vi "Button To Toggle Vr4.vi"(1 "InValue":bool, 2 "Action":enum16{"onPress", "onRelease", "Both"}(ring)) -> (0 "Result":bool)   [LabVIEW 2012]
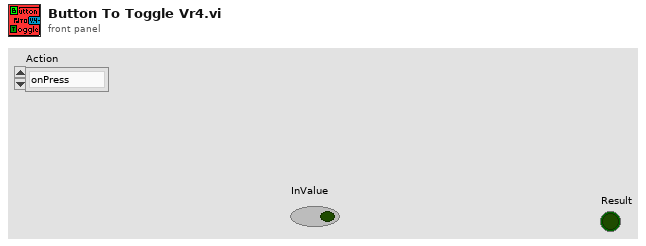
[diagram p1: front panel]
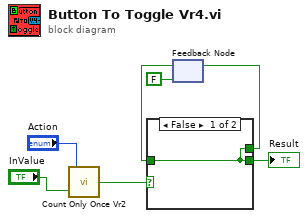
[diagram p0: block diagram]
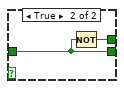
[diagram p2: hidden frame]
diagram:
  n1 = call "Count Only Once Vr2.vi"("InValue"="InValue", "Action"="Action") -> ("Result"=w2:bool)
  n2 = feedback #1(FALSE) -> (w5:bool)
  n3 = case shown="False" w2 {
    tunnel: w5 -> [w8 w9]
    tunnel: [w8 w10] -> w4
    tunnel: [w8 w9] -> w7
    frame False {
    }
    frame True {
      n4 = Not(x=w9) -> (.not. x?=w10:bool)
    }
  }
  "Result" <- w7
  n5 = feedback-in #1(w4) -> ()
